vi "Run.vi"(8 "error in (no error)":errorcluster, 11 "SimulatedBattery in":refnum<class "SimulatedBattery.lvclass">) -> (0 "error out":errorcluster, 3 "SimulatedBattery out":refnum<class "SimulatedBattery.lvclass">)   [LabVIEW 2013, in "SimulatedBattery.lvclass"]
uses:
  SimulatedBattery.lvclass
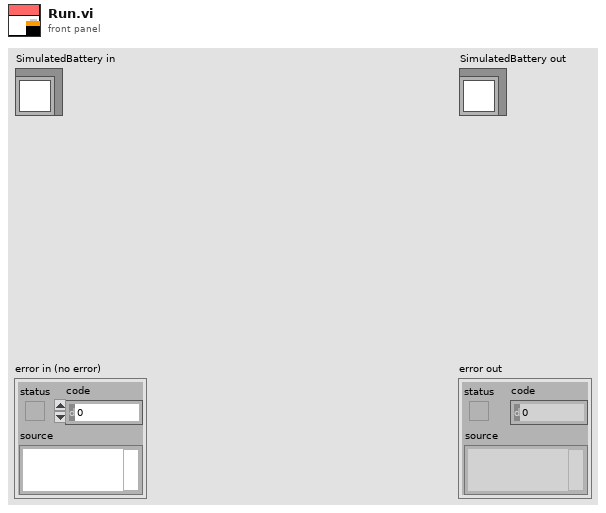
[diagram p1: front panel]
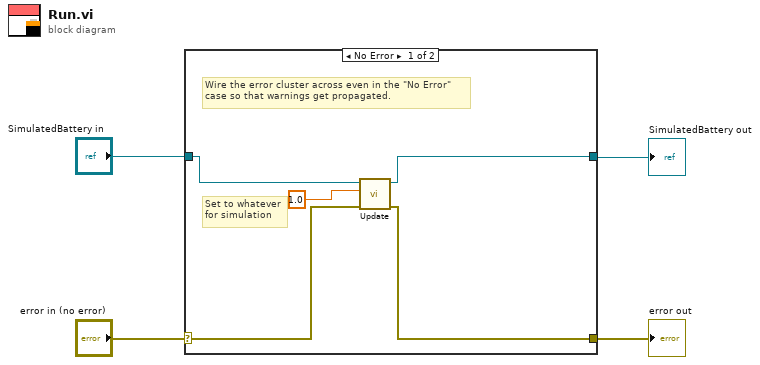
[diagram p0: block diagram]
diagram:
  n1 = case shown="No Error" "error in (no error)" {
    selector: "error in (no error)" -> [w6 w11]
    tunnel: [w5 w11] -> w1
    tunnel: [w8 w10] -> w2
    tunnel: "SimulatedBattery in" -> [w9 w10]
    frame No Error {
      # "Set to whatever\nfor simulation"
      # "Wire the error cluster across even in the \"No Error\"\ncase so that warnings get propagated."
      n2 = call-dynamic "Update.vi"("error in (no error)"=w6, "Numeric"=1.0, "AbstractBattery in"=w9) -> ("error out"=w5:errorcluster, "AbstractBattery out"=w8:refnum<class "SimulatedBattery.lvclass">)  [unwired: 7 in]
    }
    frame Error {
    }
  }
  "error out" <- w1
  "SimulatedBattery out" <- w2
